vi "logp1.vi"() -> ()   [LabVIEW 2019]
uses:
  <vilib>/Analysis/4window.llb/windowTd.ctl
  <vilib>/Instr/_visa.llb/VISA Configure Serial Port (Instr).vi
  <vilib>/measure/maspectr.llb/FFT Spectrum (Real-Im) for 1 Chan.vi
  <vilib>/Analysis/NI_AALBase.lvlib
  <vilib>/measure/NI_MAPro.lvlib
  <vilib>/Analysis/NI_AALPro.lvlib
  <vilib>/httpClient/LabVIEWHTTPClient.lvlib
panel:
  in  "Tab Control":T1(tab)
  in  "Entrer":bool
  in  "Close":bool
  in  "Reset":bool
  in  "Login":bool
  in  "Pass Word":string
  in  "User name":string
  in  "sexe":string
  in  "Age":string
  in  "nom":string
  in  "CIN":string
  in  "prenom":string
  in  "Refresh":bool
  in  "Next":bool
  in  "pas envoyer":bool
  in  "envoyer":bool
  out "body 2":string
  in  "help":bool
  in  "Lock":bool
  in  "logg":bool
  in  "Documentation EMG":bool
  in  "Precedent":bool
  in  "Analyse fréquentielle":bool
  in  "Analyse temporelle":bool
  out "?":bool
  out "nomale":string
  out "?":dbl(graph)
  out "RMS":dbl
  out "en":dbl
  out "std":dbl
  out "?":string
  in  "marche":bool
  in  "Suivant":bool
  in  "Acueil":bool
  in  "VISA resource name 3":refnum<visa-resource-name>
  in  "stop":bool
  out "mean":dbl
  out "?":bool
  out "body":string
  in  "Jump":bool
  in  "pge3":bool
  in  "help1":bool
  in  "help3":bool
  out "Spectre":dbl[](graph)
  in  "Accueil2":bool
  in  "fermer":bool
  in  "precedent2":bool
  in  "help4":bool
  in  "accueil3":bool
  in  "fermer1":bool
  in  "First":bool
  in  "First  2":bool
  in  "accueil3 2":bool
  in  "fermer1 2":bool
  # "Bienvenue"
  # "Authentification"
  # "Formulaire d'inscription"
  # "nom:"
  # "prenom:"
  # "CIN:"
  # "Age:"
  # "Sexe:"
  # "Traitement de Signal EMG"
  # "Analyse Temporelle"
  # "Les paramètres"
  # "Amplitude(uv)"
  # "Moyenne(uv)"
  # "L'écart type(uv)"
  # "L'energie(uJ)"
  # "RMS(uv)"
  # "Analyse Fréquentielle"
  # "Signal EMG"
  # "Définition"
  # "L'électromyographie (EMG) est une méthode permettant d'évaluer l'activité potentielle des unités motrices dans une région musculaire. Lorsque les potentiels d'action (signaux électriques) se propagent par les nerfs jusqu'aux jonctions neuromusculaires,  la variation des potentiels électriques (tension) peut être mesurée."
  # "EMG Brut"
  # "Remarque"
  # "-Normal : Amplitude <1mv .\n-Myopathie : Amplitude <2mV \n-Neuropathie : Amplitude >5 mV."
  # "AIDE"
  # "Pour voir le fonctionnement de  votre capteur il faut tout d'abord :\nselectionner le port com \"1\"qui'est déjà créé lorsque vous avez connceté votre carte d'acquisition puis il faut cliquer sur le bouton Power \"2\"et vous allez voir la courbe de votre signal EMG en temps réel. cette acquisition va durer une certaine période de temps puis elle va s'arrêter pour calculer les paramètres correspondants après le calcul ils vont s'afficher à droite de l'écran \"3\" et selon ses valeurs un message sera afficher au haut de la courbe (normal ou bien pathologique )\"4\"et vous pouvez vérifier si vos paramètres ont été bien envoyées vers votre base des données ou pas par le message qui s'affiche à la fin d'acquisition au dessous à droite de l'écran (\"bien :)\"si les paramètres ont été enregistées correctement si non le message \"échoué\" va être afficher) \"5\" si vous voulez voir le spectre de votre signal  il suffit de cliquer sur le flèche au haut à droite de l'écran\"7\" mais si vous voulez arrêter l'application il suffit just d'appuier sur le bouton sotp\"6\"ou bien aller vers l'acceuil à travers le bouton accueil\"8\"ou bien aller vers la page précédente\"9\"."
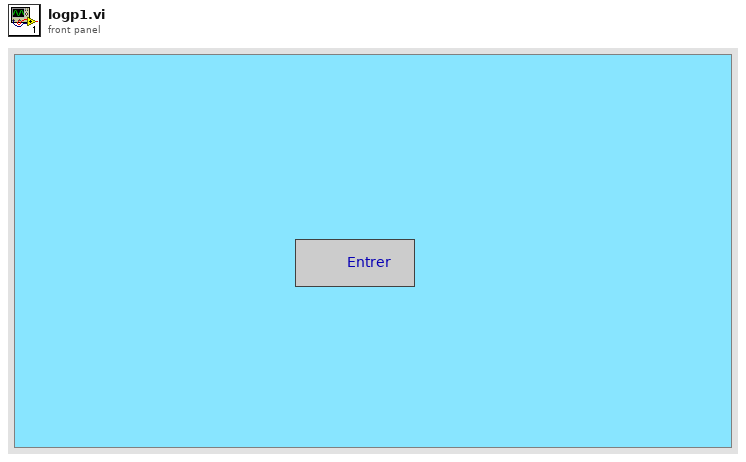
[diagram p1: front panel]
types:
  T1 = enum32{"Page 1", "Page 2", "Page 7", "Page 3", "Page 4", "Page 5", "Page 6", "Page 8"}
  T2 = enum32{"Page 1", "Page 2", "Page 7", "Page 3", "Page 4", "Page 5", "Page 6"}
  T3 = typedef "NI_AALPro.lvlib/windowTd.ctl" = u32
  T4 = cluster{"f0":dbl, "df":dbl, "imaginary part":dbl[]}
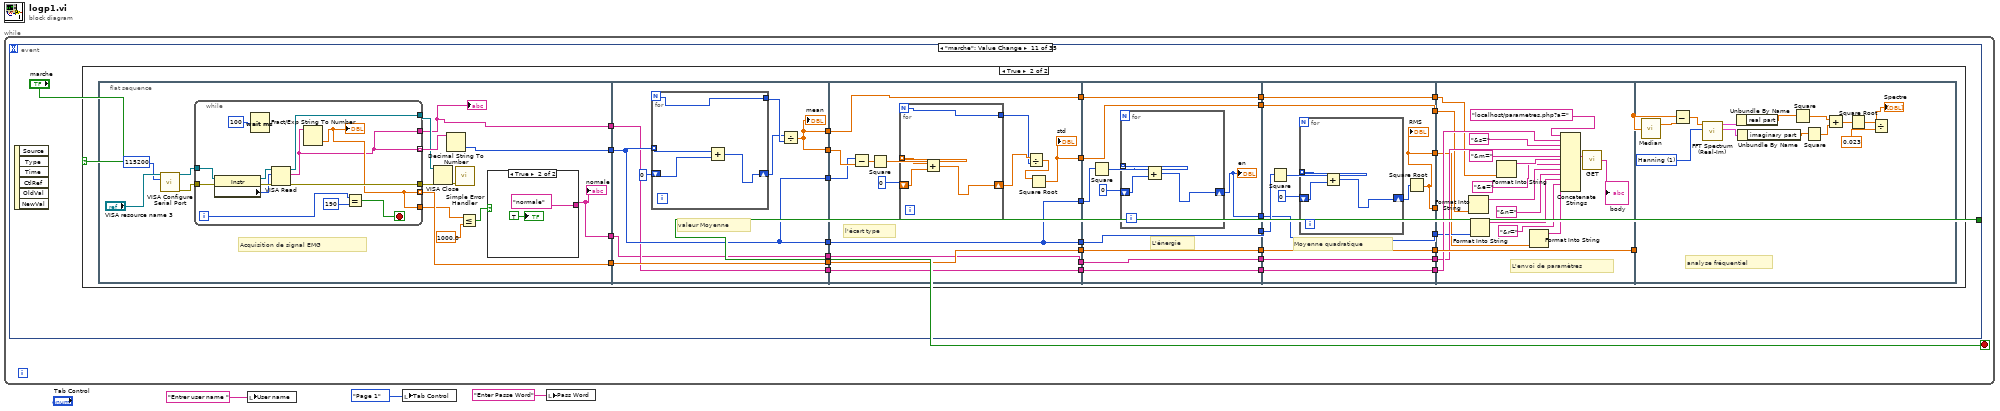
[diagram p0: block diagram]
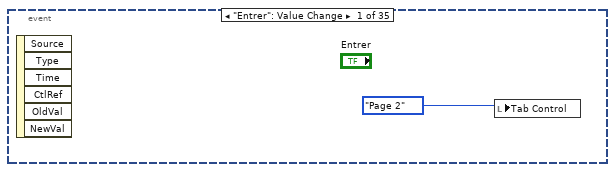
[diagram p2: hidden frame]
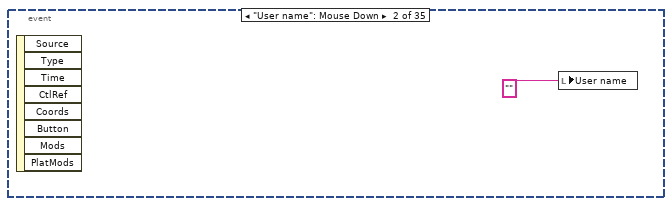
[diagram p3: hidden frame]
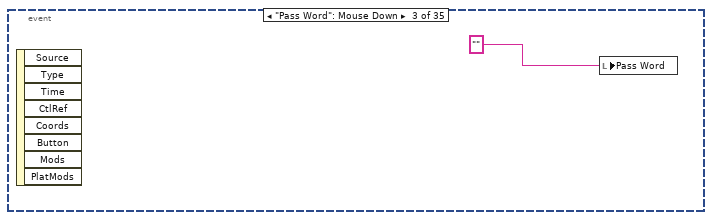
[diagram p4: hidden frame]
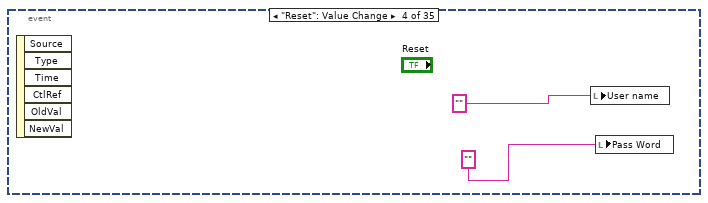
[diagram p5: hidden frame]
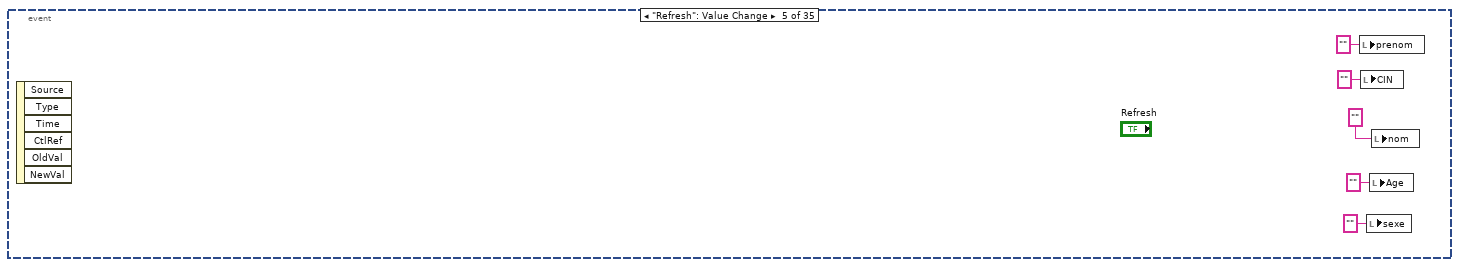
[diagram p6: hidden frame]
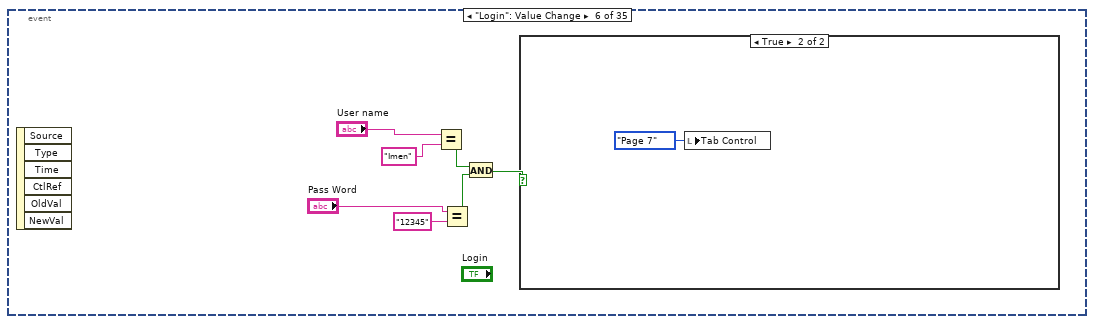
[diagram p7: hidden frame]
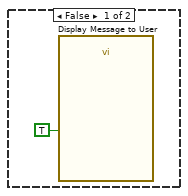
[diagram p8: hidden frame]
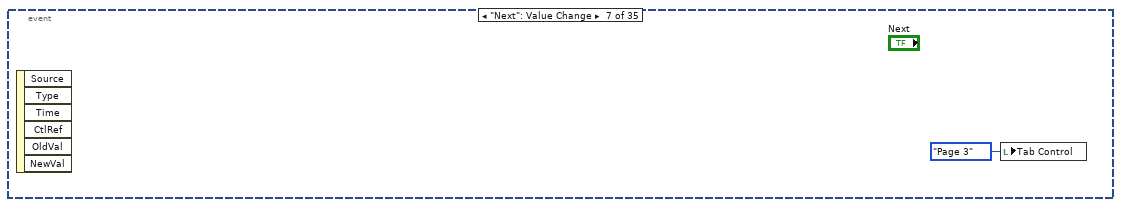
[diagram p9: hidden frame]
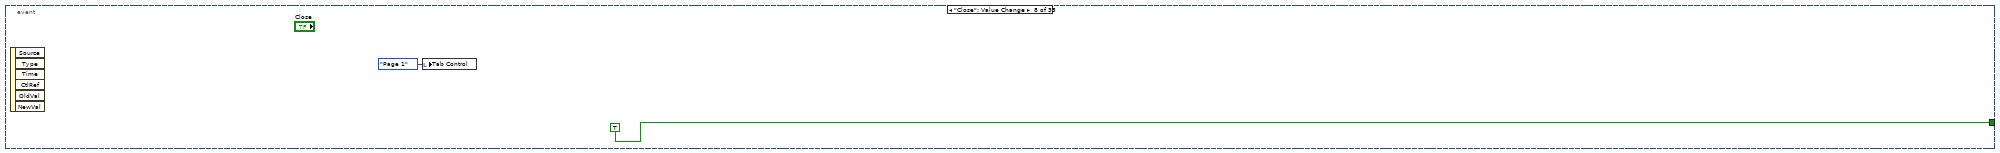
[diagram p10: hidden frame]
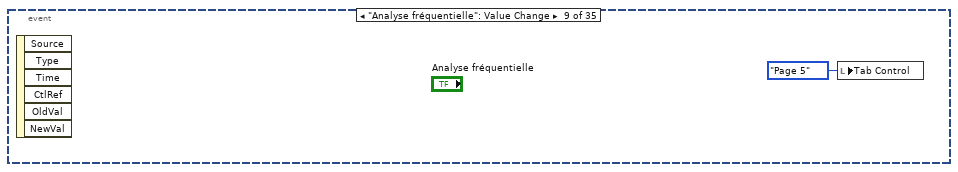
[diagram p11: hidden frame]
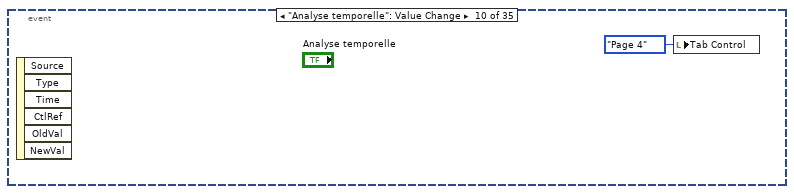
[diagram p12: hidden frame]
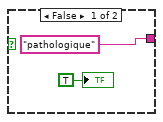
[diagram p14: hidden frame]
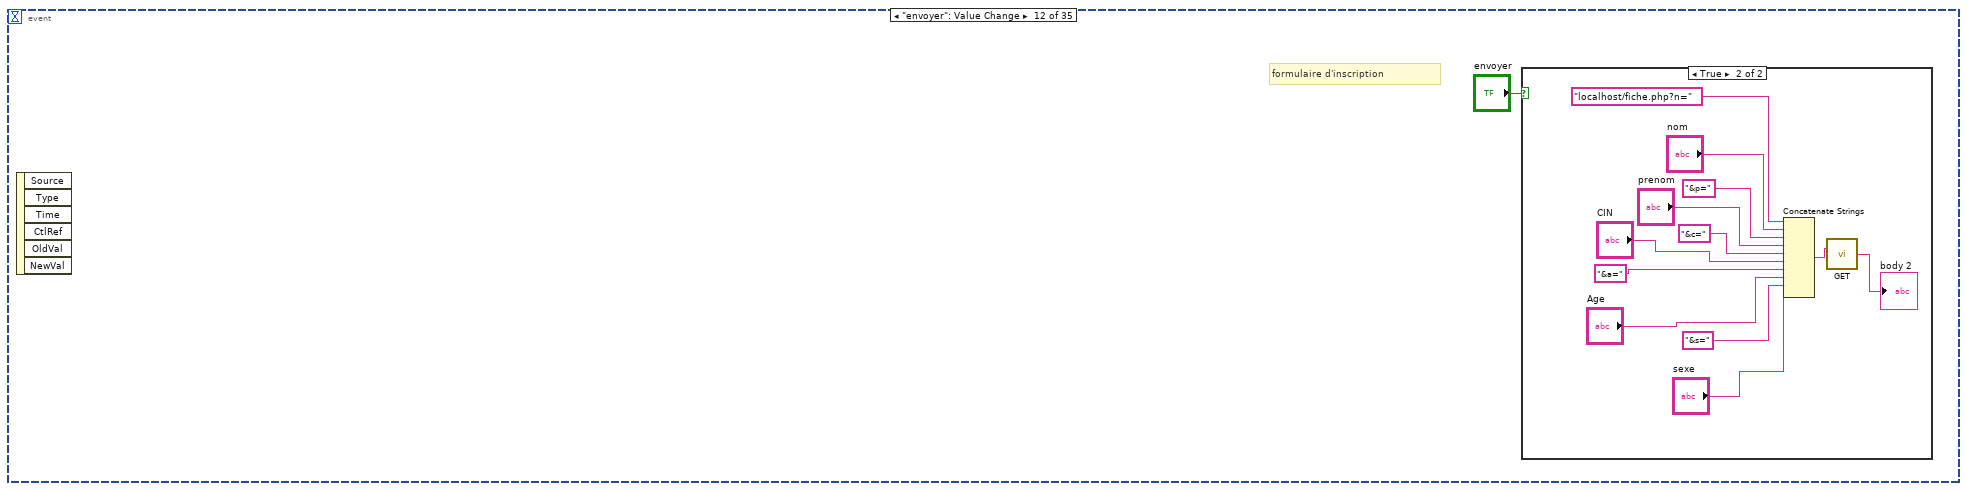
[diagram p15: hidden frame]
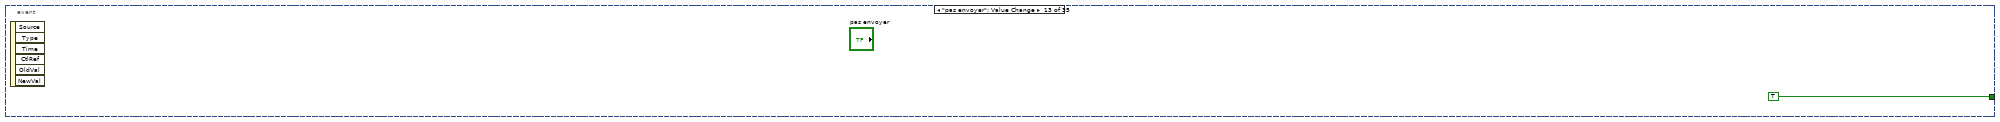
[diagram p17: hidden frame]
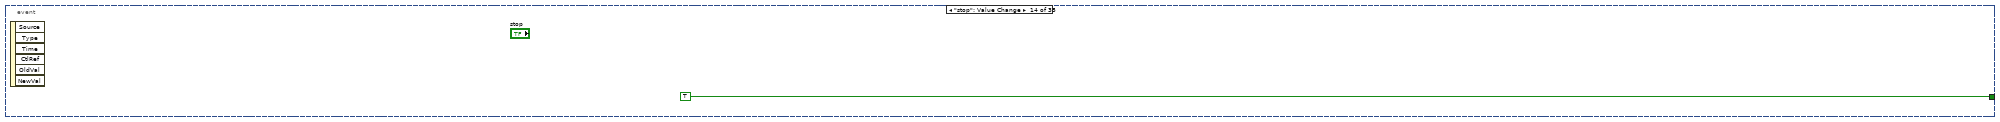
[diagram p18: hidden frame]
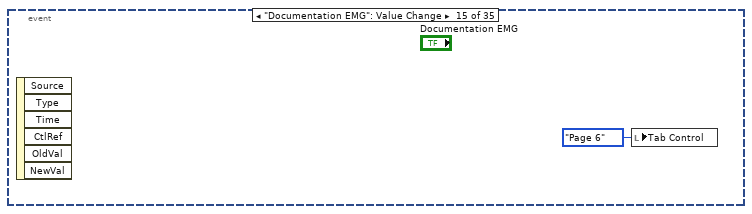
[diagram p19: hidden frame]
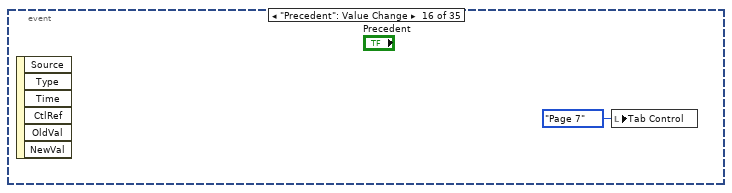
[diagram p20: hidden frame]
diagram:
  n1 = while {
    stop <- w4 stop-if-true
    n2 = event shown="[10] \"marche\": Value Change" {
      selector: _ -> [_ _ _ _ _ _ _ _ _ _ _ _ _ _ _ _ _ _ _ _ _ _ _ _ _ _ _ _ _ _ _ _ _ _ _]
      dyn-events: _ -> [_ _ _ _ _ _ _ _ _ _ _ _ _ _ _ _ _ _ _ _ _ _ _ _ _ _ _ _ _ _ _ _ _ _ _]
      timeout: _ -> [_ _ _ _ _ _ _ _ _ _ _ _ _ _ _ _ _ _ _ _ _ _ _ _ _ _ _ _ _ _ _ _ _ _ _]
      tunnel: [_ _ _ _ _ _ _ TRUE _ _ _ _ TRUE TRUE _ _ _ _ _ _ _ _ TRUE _ _ _ _ TRUE _ _ _ _ _ TRUE TRUE] -> w4
      event "Entrer": Value Change {
        n3 = event-data() -> ()  [unwired: 1 in, 6 out]
        n4 = local write "Tab Control"(enum32{"Page 1", "Page 2"}."Page 2" ("Tab Control")) -> ()
      }
      event "User name": Mouse Down {
        n5 = event-data() -> ()  [unwired: 1 in, 8 out]
        n6 = local write "User name"("" ("User name")) -> ()
      }
      event "Pass Word": Mouse Down {
        n7 = event-data() -> ()  [unwired: 1 in, 8 out]
        n8 = local write "Pass Word"("" ("Pass Word")) -> ()
      }
      event "Reset": Value Change {
        n9 = event-data() -> ()  [unwired: 1 in, 6 out]
        n10 = local write "User name"("" ("User name")) -> ()
        n11 = local write "Pass Word"("" ("Pass Word")) -> ()
      }
      event "Refresh": Value Change {
        n12 = event-data() -> ()  [unwired: 1 in, 6 out]
        n13 = local write "prenom"("" ("prenom")) -> ()
        n14 = local write "CIN"("" ("CIN")) -> ()
        n15 = local write "sexe"("" ("sexe")) -> ()
        n16 = local write "Age"("" ("Age")) -> ()
        n17 = local write "nom"("" ("nom")) -> ()
      }
      event "Login": Value Change {
        n18 = event-data() -> ()  [unwired: 1 in, 6 out]
        n19 = Equal?(x="User name", y="Imen") -> (x = y?=w20:bool)
        n20 = Equal?(x="Pass Word", y="12345") -> (x = y?=w19:bool)
        n21 = And(x=w20, y=w19) -> (x .and. y?=w15:bool)
        n22 = case shown="True" w15 {
          frame False {
            n23 = call "Display Message to User"("Enable"=TRUE) -> ()  [unwired: 9 in, 2 out]
          }
          frame True {
            n24 = local write "Tab Control"(T2."Page 7" ("Tab Control")) -> ()
          }
        }
      }
      event "Next": Value Change {
        n25 = event-data() -> ()  [unwired: 1 in, 6 out]
        n26 = local write "Tab Control"(T2."Page 3" ("Tab Control")) -> ()
      }
      event "Close": Value Change {
        n27 = event-data() -> ()  [unwired: 1 in, 6 out]
        n28 = local write "Tab Control"(T2."Page 1" ("Tab Control")) -> ()
      }
      event "Analyse fréquentielle": Value Change {
        n29 = event-data() -> ()  [unwired: 1 in, 6 out]
        n30 = local write "Tab Control"(T2."Page 5" ("Tab Control")) -> ()
      }
      event "Analyse temporelle": Value Change {
        n31 = event-data() -> ()  [unwired: 1 in, 6 out]
        n32 = local write "Tab Control"(T2."Page 4" ("Tab Control")) -> ()
      }
      event "marche": Value Change {
        n33 = event-data() -> ()  [unwired: 1 in, 6 out]
        n34 = case shown="True" "marche" {
          frame False {
          }
          frame True {
            n35 = flat-sequence {
              tunnel: [w72] -> w63
              tunnel: [w71] -> w58
              tunnel: [w64] -> w50
              tunnel: [w66] -> w35
              tunnel: w63 -> [w100]
              tunnel: [w97] -> w62
              tunnel: [w100] -> w61
              tunnel: [w100] -> w59
              tunnel: w58 -> [w99]
              tunnel: [w99] -> w57
              tunnel: w50 -> [w98]
              tunnel: [w98] -> w46
              tunnel: [w97] -> w45
              tunnel: w35 -> [w96]
              tunnel: [w96] -> w33
              tunnel: w62 -> [w120]
              tunnel: w61 -> [w116]
              tunnel: [w114] -> w60
              tunnel: w59 -> [w114]
              tunnel: w57 -> [w115]
              tunnel: [w115] -> w56
              tunnel: [w114] -> w53
              tunnel: [w113] -> w47
              tunnel: w46 -> [w113]
              tunnel: w45 -> [w112]
              tunnel: [w112] -> w42
              tunnel: [w111] -> w39
              tunnel: [w110] -> w34
              tunnel: w33 -> [w110]
              tunnel: w60 -> [w133]
              tunnel: w56 -> [w132]
              tunnel: [w132] -> w55
              tunnel: [w131] -> w54
              tunnel: w53 -> [w131]
              tunnel: [w130] -> w48
              tunnel: w47 -> [w130]
              tunnel: [w129] -> w43
              tunnel: w42 -> [w129]
              tunnel: [w128] -> w40
              tunnel: w39 -> [w128]
              tunnel: [w127] -> w38
              tunnel: w34 -> [w126]
              tunnel: [w126] -> w31
              tunnel: w55 -> [w149]
              tunnel: [w149] -> w52
              tunnel: w54 -> [w145]
              tunnel: [w144] -> w49
              tunnel: w48 -> [w144]
              tunnel: [w143] -> w44
              tunnel: w43 -> [w143]
              tunnel: [w142] -> w41
              tunnel: w40 -> [w142]
              tunnel: w38 -> [w141]
              tunnel: [w141] -> w37
              tunnel: [w139] -> w36
              tunnel: [w140] -> w32
              tunnel: w31 -> [w140]
              tunnel: [w139] -> w30
              tunnel: w52 -> [w171]
              tunnel: [w171] -> w51
              tunnel: w49 -> [w169]
              tunnel: w44 -> [w164]
              tunnel: w41 -> [w161]
              tunnel: w37 -> [w158]
              tunnel: w36 -> [_]
              tunnel: w32 -> [w166]
              tunnel: w30 -> [w154]
              tunnel: w51 -> [w185]
              frame #0 {
                # "Acquisition de signal EMG"
                n36 = call-poly "VISA Configure Serial Port"("VISA resource name"="VISA resource name 3", "baud rate (9600)"=u32 115200 ("timeout (10sec)")) -> ("VISA resource name out"=w74:refnum<visa-resource-name>, "error out"=w75:errorcluster)  [unwired: 12 in]
                n37 = while {
                  tunnel: w74 -> [w95]
                  tunnel: w75 -> [w94]
                  tunnel: [w90] -> w78
                  tunnel: [w89] -> w67
                  tunnel: [w83] -> w73 mode=indexing
                  tunnel: [w84] -> w71 mode=indexing
                  tunnel: [w84] -> w70
                  tunnel: [w83] -> w64
                  i -> [w87]
                  stop <- w85 stop-if-true
                  n38 = property class="Instr"(reference=w95, error in=w94) -> (reference out=w92:refnum<visa-resource-name>, error out=w93:errorcluster, "Serial Settings:Number of Bytes at Serial Port"=w91:u32)
                  n39 = Wait (ms)(milliseconds to wait=u32 100) -> ()  [unwired: 1 out]
                  n40 = VISA Read(VISA resource name=w92, byte count=w91, error in (no error)=w93) -> (VISA resource name out=w89:refnum<visa-resource-name>, read buffer=w83:string, error out=w90:errorcluster)  [unwired: 1 out]
                  n41 = Fract/Exp String To Number(string=w83) -> (number=w84:dbl)  [unwired: 3 in, 1 out]
                  "?" <- w84
                  n42 = Equal?(x=w87, y=190) -> (x = y?=w85:bool)
                }
                "?" <- w64
                n43 = VISA Close(VISA resource name=w67, error in (no error)=w78) -> (error out=w77:errorcluster)
                n44 = Decimal String To Number(string=w73) -> (number=w72:i32[])  [unwired: 2 in, 1 out]
                n45 = call <vilib>:"Simple Error Handler.vi"("error in (no error)"=w77) -> ()  [unwired: 4 in, 5 out]
                n46 = Less Or Equal?(x=w70, y=1000.0) -> (x <= y?=w68:bool)
                n47 = case shown="True" w68 {
                  tunnel: ["pathologique" ("nomale") "normale" ("nomale")] -> w66
                  frame False {
                    "?" <- TRUE
                  }
                  frame True {
                    "?" <- TRUE ("normale")
                  }
                }
                "nomale" <- w66
              }
              frame #1 {
                # "valeur Moyenne"
                n48 = for {
                  N -> [w105]
                  shift-right: [w106] -> w101
                  shift-left: 0 -> [w107]
                  tunnel: [w105] -> w103
                  tunnel: w100 -> [w104] mode=indexing
                  n49 = Add(x=w104, y=w107) -> (x+y=w106:i32)
                }
                n50 = Divide(x=w101, y=w103) -> (x/y=w97:dbl)
                "mean" <- w97
              }
              frame #2 {
                # "l'écart type"
                n51 = Subtract(x=w116, y=w120) -> (x-y=w121:dbl[])
                n52 = Square(x=w121) -> (x^2=w119:dbl[])
                n53 = for {
                  N -> [w122]
                  shift-right: [w125] -> w109
                  shift-left: 0 -> [w123]
                  tunnel: w119 -> [w124] mode=indexing
                  tunnel: [w122] -> w108
                  n54 = Add(x=w124, y=w123) -> (x+y=w125:dbl)
                }
                n55 = Divide(x=w109, y=w108) -> (x/y=w117:dbl)
                n56 = Square Root(x=w117) -> (sqrt(x)=w111:dbl)
                "std" <- w111
              }
              frame #3 {
                # "L'énergie"
                n57 = Square(x=w133) -> (x^2=w134:i32[])
                n58 = for {
                  shift-right: [w138] -> w127
                  shift-left: 0 -> [w136]
                  tunnel: w134 -> [w137] mode=indexing
                  n59 = Add(x=w137, y=w136) -> (x+y=w138:i32)
                }
                "en" <- w127
              }
              frame #4 {
                # "Moyenne quadratique"
                n60 = Square(x=w145) -> (x^2=w148:i32[])
                n61 = for {
                  shift-right: [w152] -> w146
                  shift-left: 0 -> [w150]
                  tunnel: w148 -> [w151] mode=indexing
                  n62 = Add(x=w151, y=w150) -> (x+y=w152:i32)
                }
                n63 = Square Root(x=w146) -> (sqrt(x)=w139:dbl)
                "RMS" <- w139
              }
              frame #5 {
                # "L'envoi de paramètres"
                n64 = Format Into String(w161) -> (resulting string=w159:string)  [unwired: 3 in, 1 out]
                n65 = Format Into String(w158) -> (resulting string=w155:string)  [unwired: 3 in, 1 out]
                n66 = Format Into String(w164) -> (resulting string=w162:string)  [unwired: 3 in, 1 out]
                n67 = Format Into String(w154) -> (resulting string=w153:string)  [unwired: 3 in, 1 out]
                n68 = Concatenate Strings("localhost/parametres.php?a=" ("string"), w169, "&s=" ("string"), w166, "&m=" ("string"), w162, "&e=" ("string"), w159, "&n=" ("string"), w155, "&r=" ("string"), w153) -> (w168:string)
                n69 = call <vilib>:"GET.vi"("url"=w168) -> ("body"=→"body":string)  [unwired: 11 in, 3 out]
              }
              frame #6 {
                w182 = T3 1 items=["Rectangle"=0, "Hanning"=1, "Hamming"=2, "Blackman-Harris"=3, "Exact Blackman"=4, "Blackman"=5, "Flat Top"=6, "4 Term B-Harris "=7, "7 Term B-Harris"=8, "Low Sidelobe"=9, "Blackman Nuttall"=11, "Triangle"=30, "Bartlett-Hanning"=31, "Bohman"=32, "Parzen"=33, "Welch"=34, "Kaiser"=60, "Dolph-Chebyshev"=61, "Gaussian"=62] ("window")
                # "analyse fréquentiel"
                n70 = call <vilib>:"Median.vi"("X"=w185) -> ("median"=w184:dbl)  [unwired: 1 out]
                n71 = Subtract(x=w185, y=w184) -> (x-y=w183:dbl[])
                n72 = call-poly <vilib>:"FFT Spectrum (Real-Im).vi"("window"=w182, "time signal"=w183) -> ("imaginary part"=w180:T4, "real part"=w181:cluster{"f0":dbl, "df":dbl, "real part":dbl[]})  [unwired: 5 in, 3 out]
                n73 = Unbundle By Name(w181) -> ("real part"=w179:dbl[])
                n74 = Unbundle By Name(w180) -> ("imaginary part"=w178:dbl[])
                n75 = Square(x=w179) -> (x^2=w176:dbl[])
                n76 = Square(x=w178) -> (x^2=w177:dbl[])
                n77 = Add(x=w176, y=w177) -> (x+y=w175:dbl[])
                n78 = Square Root(x=w175) -> (sqrt(x)=w174:dbl[])
                n79 = Divide(x=w174, y=0.023) -> (x/y=→"Spectre":dbl[])
              }
            }
          }
        }
      }
      event "envoyer": Value Change {
        # "formulaire d'inscription"
        n80 = event-data() -> ()  [unwired: 1 in, 6 out]
        n81 = case shown="True" "envoyer" {
          frame False {
          }
          frame True {
            n82 = Concatenate Strings("localhost/fiche.php?n=" ("string"), "nom", "&p=" ("string"), "prenom", "&c=" ("string"), "CIN", "&a=" ("string"), "Age", "&s=" ("string"), "sexe") -> (w188:string)
            n83 = call <vilib>:"GET.vi"("url"=w188) -> ("body"=→"body 2":string)  [unwired: 11 in, 3 out]
          }
        }
      }
      event "pas envoyer": Value Change {
        n84 = event-data() -> ()  [unwired: 1 in, 6 out]
      }
      event "stop": Value Change {
        n85 = event-data() -> ()  [unwired: 1 in, 6 out]
      }
      event "Documentation EMG": Value Change {
        n86 = event-data() -> ()  [unwired: 1 in, 6 out]
        n87 = local write "Tab Control"(T2."Page 6" ("Tab Control")) -> ()
      }
      event "Precedent": Value Change {
        n88 = event-data() -> ()  [unwired: 1 in, 6 out]
        n89 = local write "Tab Control"(T2."Page 7" ("Tab Control")) -> ()
      }
      event "First": Value Change {
        n90 = event-data() -> ()  [unwired: 1 in, 6 out]
        n91 = local write "Tab Control"(T2."Page 3" ("Tab Control")) -> ()
      }
      event "Jump": Value Change {
        n92 = event-data() -> ()  [unwired: 1 in, 6 out]
        n93 = local write "Tab Control"(T2."Page 6" ("Tab Control")) -> ()
      }
      event "pge3": Value Change {
        n94 = event-data() -> ()  [unwired: 1 in, 6 out]
        n95 = local write "Tab Control"(T2."Page 3" ("Tab Control")) -> ()
      }
      event "logg": Value Change {
        n96 = event-data() -> ()  [unwired: 1 in, 6 out]
        n97 = local write "Tab Control"(T2."Page 2" ("Tab Control")) -> ()
      }
      event "Acueil": Value Change {
        n98 = event-data() -> ()  [unwired: 1 in, 6 out]
        n99 = local write "Tab Control"(T2."Page 7" ("Tab Control")) -> ()
      }
      event "Suivant": Value Change {
        n100 = event-data() -> ()  [unwired: 1 in, 6 out]
        n101 = local write "Tab Control"(T2."Page 5" ("Tab Control")) -> ()
      }
      event "Lock": Value Change {
        n102 = event-data() -> ()  [unwired: 1 in, 6 out]
        n103 = local write "Tab Control"(T2."Page 1" ("Tab Control")) -> ()
      }
      event "precedent2": Value Change {
        n104 = event-data() -> ()  [unwired: 1 in, 6 out]
        n105 = local write "Tab Control"(T2."Page 4" ("Tab Control")) -> ()
      }
      event "Accueil2": Value Change {
        n106 = event-data() -> ()  [unwired: 1 in, 6 out]
        n107 = local write "Tab Control"(T2."Page 7" ("Tab Control")) -> ()
      }
      event "accueil3 2": Value Change {
        n108 = event-data() -> ()  [unwired: 1 in, 6 out]
        n109 = local write "Tab Control"(T1."Page 7" ("Tab Control")) -> ()
      }
      event "First  2": Value Change {
        n110 = event-data() -> ()  [unwired: 1 in, 6 out]
        n111 = local write "Tab Control"(T1."Page 3" ("Tab Control")) -> ()
      }
      event "fermer": Value Change {
        n112 = event-data() -> ()  [unwired: 1 in, 6 out]
        n113 = local write "Tab Control"(T2."Page 1" ("Tab Control")) -> ()
      }
      event "accueil3": Value Change {
        n114 = event-data() -> ()  [unwired: 1 in, 6 out]
        n115 = local write "Tab Control"(T2."Page 7" ("Tab Control")) -> ()
      }
      event "help": Value Change {
        n116 = event-data() -> ()  [unwired: 1 in, 6 out]
        n117 = local write "Tab Control"(T1."Page 8" ("Tab Control")) -> ()
      }
      event "help1": Value Change {
        n118 = event-data() -> ()  [unwired: 1 in, 6 out]
        n119 = local write "Tab Control"(T1."Page 8" ("Tab Control")) -> ()
      }
      event "help3": Value Change {
        n120 = event-data() -> ()  [unwired: 1 in, 6 out]
        n121 = local write "Tab Control"(T1."Page 8" ("Tab Control")) -> ()
      }
      event "help4": Value Change {
        n122 = event-data() -> ()  [unwired: 1 in, 6 out]
        n123 = local write "Tab Control"(T1."Page 8" ("Tab Control")) -> ()
      }
      event "fermer1": Value Change {
        n124 = event-data() -> ()  [unwired: 1 in, 6 out]
        n125 = local write "Tab Control"(T2."Page 1" ("Tab Control")) -> ()
      }
      event "fermer1 2": Value Change {
        n126 = event-data() -> ()  [unwired: 1 in, 6 out]
      }
    }
  }
  n127 = local write "User name"("Entrer user name " ("User name")) -> ()
  n128 = local write "Tab Control"(enum32{"Page 1", "Page 2"}."Page 1" ("Tab Control")) -> ()
  n129 = local write "Pass Word"("Enter Passe Word" ("Pass Word")) -> ()
